vi "Row-Col Processing.vi"(5 "Array bounds":cluster{"Max X":i16, "Max Y":i16}, 7 "Penetration":i16, 8 "Row/Col to test":i16, 10 "Side":enum16{"Top", "Left", "Bottom", "Right"}(ring)) -> (0 "Last Row/Column?":bool, 1 "Done?":bool, 2 "X":i16, 3 "Y":i16)   [LabVIEW 2012]
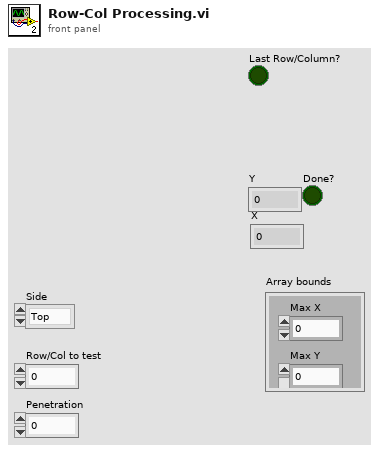
[diagram p1: front panel]
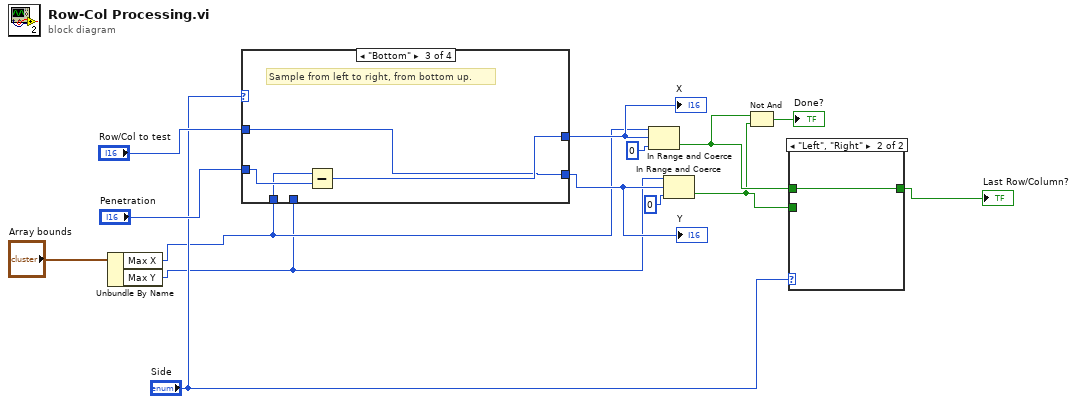
[diagram p0: block diagram]
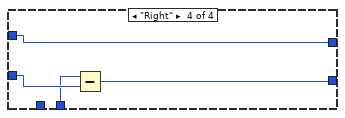
[diagram p5: hidden frame]
diagram:
  n1 = Unbundle By Name("Array bounds") -> ("Max X"=w2:i16, "Max Y"=w1:i16)
  n2 = case shown="\"Bottom\"" "Side" {
    tunnel: "Row/Col to test" -> [w15 w17 w20 w24]
    tunnel: "Penetration" -> [w16 w18 w22 w26]
    tunnel: [w16 w17 w20 w25] -> w8
    tunnel: [w15 w18 w21 w24] -> w9
    tunnel: w1 -> [_ _ _ w23]
    tunnel: w2 -> [_ _ w19 _]
    frame "Top", Default {
      # "Move from left to right, sampling down."
    }
    frame "Left" {
      # "Move from top to bottom, sampling left to right."
    }
    frame "Bottom" {
      # "Sample from left to right, from bottom up."
      n3 = Subtract(x=w19, y=w22) -> (x-y=w21:i16)
    }
    frame "Right" {
      n4 = Subtract(x=w23, y=w26) -> (x-y=w25:i16)
    }
  }
  "Y" <- w8
  "X" <- w9
  n5 = In Range and Coerce(upper limit=w2, x=w9, lower limit=i16 0) -> (In Range?=w7:bool)  [unwired: 1 out]
  n6 = In Range and Coerce(upper limit=w1, x=w8, lower limit=i16 0) -> (In Range?=w6:bool)  [unwired: 1 out]
  n7 = Not And(1:w6, 2:w7) -> (0:→"Done?":bool)
  n8 = case shown="\"Left\", \"Right\"" "Side" {
    tunnel: w7 -> [_ w28]
    tunnel: w6 -> [w27 _]
    tunnel: [w27 w28] -> w4
    frame "Top", "Bottom" {
    }
    frame "Left", "Right" {
    }
  }
  "Last Row/Column?" <- w4
